vi "Sort Circle Center.vi"(11 "Array 3":T1(array[cluster])) -> (2 "Circle Plots":cluster{"Points":cluster{dbl, dbl}[]}[](array[cluster]), 3 "Circle Combos":T2(array[cluster]))   [LabVIEW 2025]
uses:
  9e152e3b-3a92-4c6e-af5c-e7a27942db98.vi
  9e152e3b-3a92-4c6e-af5c-e7a27942db98.vi/4611cae3-c7be-41e2-9a5e-ea0ae78a7ced.vi
  9e152e3b-3a92-4c6e-af5c-e7a27942db98.vi/4611cae3-c7be-41e2-9a5e-ea0ae78a7ced.vi/19e2e4cb-e3bb-4239-bd5f-680916605f5d.vi
  9e152e3b-3a92-4c6e-af5c-e7a27942db98.vi/4611cae3-c7be-41e2-9a5e-ea0ae78a7ced.vi/f72612c1-738a-48a1-9fcf-3db66cb27fb3.vi
  9e152e3b-3a92-4c6e-af5c-e7a27942db98.vi/4611cae3-c7be-41e2-9a5e-ea0ae78a7ced.vi/45406051-8994-464b-8b47-ac12a8cbadfa.vi
  9e152e3b-3a92-4c6e-af5c-e7a27942db98.vi/4611cae3-c7be-41e2-9a5e-ea0ae78a7ced.vi/dd886480-778c-48b1-8e4a-d6890e1a60dd.vi
  9e152e3b-3a92-4c6e-af5c-e7a27942db98.vi/4611cae3-c7be-41e2-9a5e-ea0ae78a7ced.vi/2e6e140f-e361-4312-a09e-e37273ac7fd1.vi
  9e152e3b-3a92-4c6e-af5c-e7a27942db98.vi/4611cae3-c7be-41e2-9a5e-ea0ae78a7ced.vi/3589548e-4c68-4568-af05-72ab28470577.vi
  9e152e3b-3a92-4c6e-af5c-e7a27942db98.vi/4611cae3-c7be-41e2-9a5e-ea0ae78a7ced.vi/cf64d4f5-91bd-4749-9577-68c6ded0155b.vi
  9e152e3b-3a92-4c6e-af5c-e7a27942db98.vi/4611cae3-c7be-41e2-9a5e-ea0ae78a7ced.vi/6f6fefe9-f25b-4595-b26f-75715299a794.vi
  9e152e3b-3a92-4c6e-af5c-e7a27942db98.vi/4611cae3-c7be-41e2-9a5e-ea0ae78a7ced.vi/c74ffb76-1048-4639-9a95-b6de96ba7014.vi
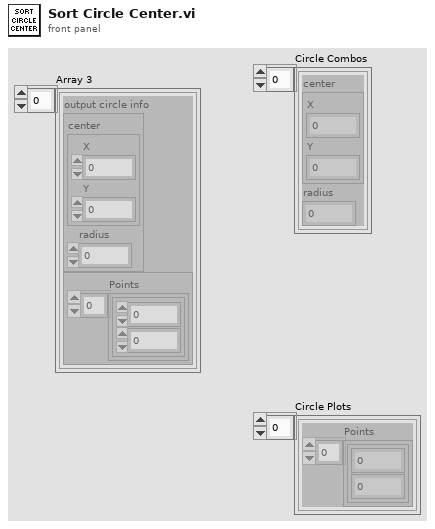
[diagram p1: front panel]
types:
  T1 = cluster{"output circle info":cluster{"center":cluster{"X":sgl, "Y":sgl}, "radius":sgl}, cluster{"Points":cluster{dbl, dbl}[]}}[]
  T2 = cluster{"center":cluster{"X":sgl, "Y":sgl}, "radius":sgl}[]
  T3 = cluster{"output circle info":cluster{"center":cluster{"X":sgl, "Y":sgl}, "radius":sgl}, cluster{"Points":cluster{dbl, dbl}[]}}
  T4 = cluster{cluster{"output circle info":cluster{"center":cluster{"X":sgl, "Y":sgl}, "radius":sgl}, cluster{"Points":cluster{dbl, dbl}[]}}, cluster{"output circle info":cluster{"center":cluster{"X":sgl, "Y":sgl}, "radius":sgl}, cluster{"Points":cluster{dbl, dbl}[]}}, cluster{"output circle info":cluster{"center":cluster{"X":sgl, "Y":sgl}, "radius":sgl}, cluster{"Points":cluster{dbl, dbl}[]}}}
  T5 = cluster{cluster{"output circle info":cluster{"center":cluster{"X":sgl, "Y":sgl}, "radius":sgl}, cluster{"Points":cluster{dbl, dbl}[]}}, cluster{"output circle info":cluster{"center":cluster{"X":sgl, "Y":sgl}, "radius":sgl}, cluster{"Points":cluster{dbl, dbl}[]}}, cluster{"output circle info":cluster{"center":cluster{"X":sgl, "Y":sgl}, "radius":sgl}, cluster{"Points":cluster{dbl, dbl}[]}}}[]
  T6 = cluster{"center":cluster{"X":sgl, "Y":sgl}, "radius":sgl}
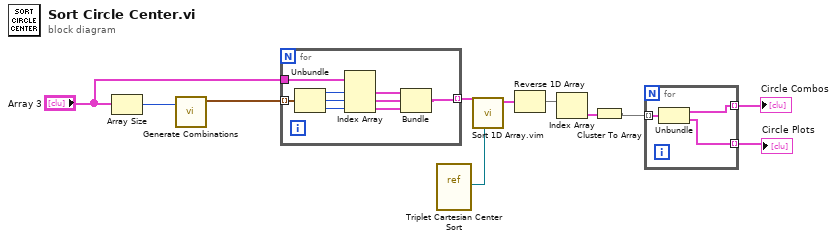
[diagram p0: block diagram]
diagram:
  n1 = Array Size(array="Array 3") -> (size(s)=w11:i32)
  n2 = call "Generate Combinations.vi"("Upper Bound"=w11) -> ("Array"=w10:cluster{i32, i32, i32}[])  [unwired: 10 in]
  n3 = for {
    tunnel: w10 -> [w19] mode=indexing
    tunnel: "Array 3" -> [w20]
    tunnel: [w12] -> w8 mode=indexing
    n4 = Unbundle(w19) -> (w18:i32, w17:i32, w16:i32)
    n5 = Index Array(array=w20, index #1=w18, index #2=w17, index #3=w16) -> (element #1=w15:T3, element #2=w14:T3, element #3=w13:T3)
    n6 = Bundle(w15, w14, w13) -> (w12:T4)  [unwired: 1 in]
  }
  n7 = vi-ref "Triplet Cartesian Center Sort.vi"() -> (w7:refnum<vi>)
  n8 = call "Sort 1D Array.vim"("less function (built-in <)"=w7, "unsorted array"=w8) -> ("sorted array"=w2:T5)  [unwired: 9 in]
  n9 = Reverse 1D Array(array=w2) -> (reversed array=w1:T5)
  n10 = Index Array(array=w1) -> (element=w6:T4)  [unwired: 1 in]
  n11 = Cluster To Array(cluster=w6) -> (array=w5:T1)
  n12 = for {
    tunnel: w5 -> [w23] mode=indexing
    tunnel: [w22] -> w4 mode=indexing
    tunnel: [w21] -> w3 mode=indexing
    n13 = Unbundle(w23) -> ("output circle info"=w22:T6, w21:cluster{"Points":cluster{dbl, dbl}[]})
  }
  "Circle Plots" <- w3
  "Circle Combos" <- w4
